vi "Max_Min Check.vi"(3 "Last Minimum":dbl, 4 "New Value":dbl, 5 "Last Maximum":dbl) -> (0 "Minimum":dbl, 2 "Maximum":dbl)   [LabVIEW 2014]
doc: "Compares new data value with the previous maximum and minimum values, and outputs the new maximum and minimum values."
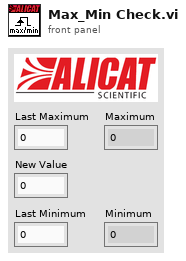
[diagram p1: front panel]
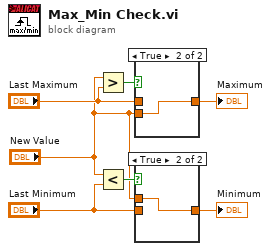
[diagram p0: block diagram]
diagram:
  n1 = Greater?(x="New Value", y="Last Maximum") -> (0:w7:bool)
  n2 = Less?(x="New Value", y="Last Minimum") -> (x < y?=w4:bool)
  n3 = case shown="True" w7 {
    tunnel: [w8 w9] -> w6
    tunnel: "New Value" -> [_ w9]
    tunnel: "Last Maximum" -> [w8 _]
    frame False {
    }
    frame True {
    }
  }
  "Maximum" <- w6
  n4 = case shown="True" w4 {
    tunnel: [w10 w11] -> w3
    tunnel: "New Value" -> [_ w11]
    tunnel: "Last Minimum" -> [w10 _]
    frame False {
    }
    frame True {
    }
  }
  "Minimum" <- w3
